vi "Untitled 5.vi"() -> ()   [LabVIEW 2017]
panel:
  out "string":string
  in  "Read Data":u8[](array[numeric])=[0, 0, 0, 0, 0, 0, 0, 0, 0, 0] format="%b"
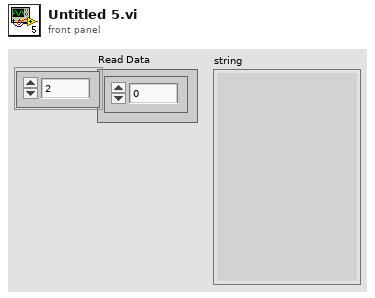
[diagram p1: front panel]
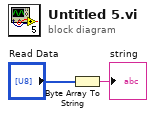
[diagram p0: block diagram]
diagram:
  n1 = Byte Array To String(unsigned byte array="Read Data") -> (string=→"string":string)
